vi "Write Word Over 2 Addresses.vi"(0 "VISA resource name":refnum<visa-resource-name>, 5 "Motor ID (0)":u8, 7 "Address number (0)":u8, 9 "Parameter (0)":u16, 11 "error in (no error)":errorcluster) -> (4 "VISA resource name out":refnum<visa-resource-name>, 15 "error out":errorcluster)   [LabVIEW 2016, in "Dynamixel Motor.lvlib"]
doc: "Writes a word type (U16) over two addresses in the motor's register. The data is written in little endian byte order. This is a Low-Level VI that is used by other VIs."
uses:
  Dynamixel Motor.lvlib
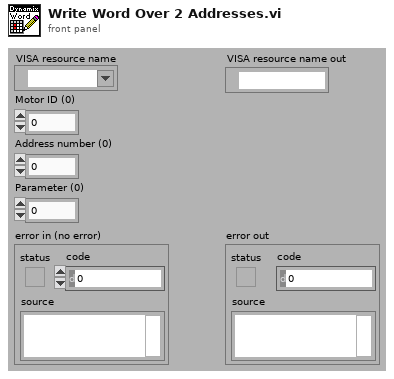
[diagram p1: front panel]
types:
  T1 = enum16{"big-endian, network order", "native, host order", "little-endian"}
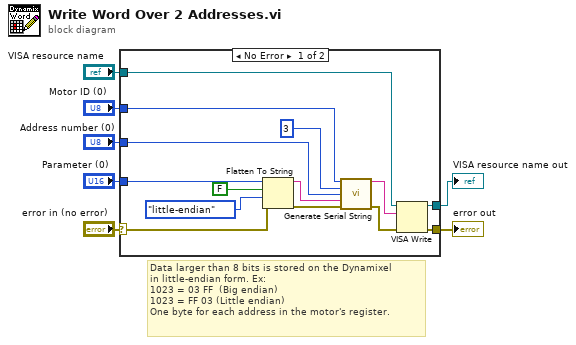
[diagram p0: block diagram]
diagram:
  # "Data larger than 8 bits is stored on the Dynamixel \nin little-endian form. Ex:\n1023 = 03 FF  (Big endian)\n1023 = FF 03 (Little endian)\nOne byte for each address in the motor's register."
  n1 = case shown="No Error" "error in (no error)" {
    selector: "error in (no error)" -> [w9 w23]
    tunnel: "Address number (0)" -> [w15 _]
    tunnel: "Motor ID (0)" -> [w17 _]
    tunnel: "VISA resource name" -> [w21 w22]
    tunnel: "Parameter (0)" -> [w14 _]
    tunnel: [w19 w22] -> w3
    tunnel: [w18 w23] -> w2
    frame No Error {
      n2 = Flatten To String(anything=w14, prepend array or string size? (T)=FALSE, byte order (0:big-endian, network order)=T1."little-endian", error in (no error)=w9) -> (data string=w13:string, error out=w8:errorcluster)  [unwired: 1 out]
      n3 = call "Generate Serial String.vi"("Motor ID"=w17, "Command"=u8 3, "Address"=w15, "Parameters"=w13, "Error in (no error)"=w8) -> ("Command to Serial"=w20:string, "error out"=w12:errorcluster)  [unwired: 9 in]
      n4 = VISA Write(VISA resource name=w21, write buffer=w20, error in (no error)=w12) -> (VISA resource name out=w19:refnum<visa-resource-name>, error out=w18:errorcluster)  [unwired: 1 out]
    }
    frame Error {
    }
  }
  "VISA resource name out" <- w3
  "error out" <- w2
